vi "LatchBooleanKeyboardSimulation_Tests.vi"(11 "error in (no error)":errorcluster) -> (15 "error out":errorcluster)   [LabVIEW 2016, in "DronaTest.lvlib"]
uses:
  DronaTest.lvlib
  APIs/Stimulus/ControlValue/ValueSignalLatchBooleanString.vi
  APIs/Assert/AssertControlValue/Equal.vi
  <vilib>/addons/_JKI Toolkits/Caraya/classes/Test/Test.lvclass
  Drona.lvlib
  APIs/Assert/AssertControlValue/AssertControlValue.lvlib
  APIs/Stimulus/ControlValue/ControlValue.lvlib
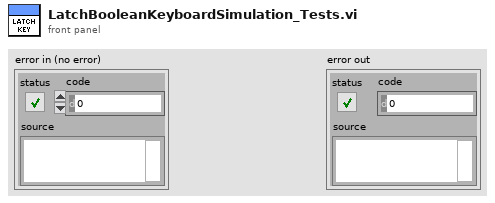
[diagram p1: front panel]
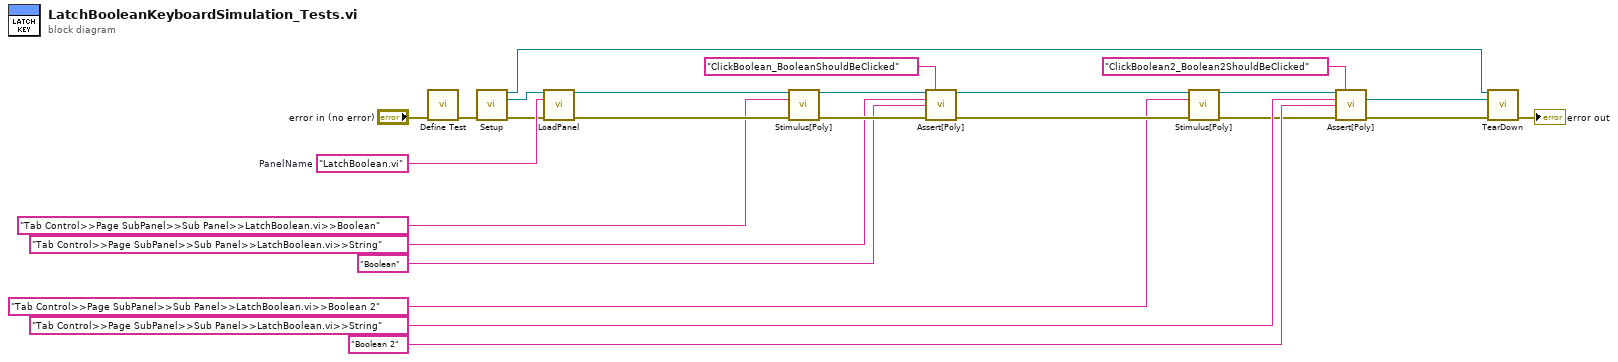
[diagram p0: block diagram]
diagram:
  w24 = "LatchBoolean.vi"  # PanelName
  n1 = call <vilib>:"Define Test.vi"("error in (no error)"="error in (no error)") -> ("error out"=w6:errorcluster)  [unwired: 10 in]
  n2 = call "Setup.vi"("error in (no error)"=w6) -> ("Application Ref"=w4:refnum<vi>, "VI out"=w2:refnum<vi>, "error out"=w3:errorcluster)  [unwired: 12 in]
  n3 = call "LoadPanel.vi"("VI in"=w2, "Panel Name"=w24, "error in (no error)"=w3) -> ("VI out"=w22:refnum<vi>, "error out"=w9:errorcluster)  [unwired: 11 in]
  n4 = call-poly "Stimulus[Poly].vi"("VI Reference In"=w22, "Control Path"="Tab Control>>Page SubPanel>>Sub Panel>>LatchBoolean.vi>>Boolean", "error in"=w9) -> ("VI Reference Out"=w21:refnum<vi>, "error out"=w23:errorcluster)  [unwired: 11 in]
  n5 = call-poly "Assert[Poly].vi"("VI Reference In"=w21, "Test Label"="ClickBoolean_BooleanShouldBeClicked" ("string"), "Control Path"="Tab Control>>Page SubPanel>>Sub Panel>>LatchBoolean.vi>>String", "Control Value"="Boolean" ("Control Path"), "Error In"=w23) -> ("VI Reference Out"=w11:refnum<vi>, "Error Out"=w12:errorcluster)  [unwired: 9 in]
  n6 = call-poly "Stimulus[Poly].vi"("VI Reference In"=w11, "Control Path"="Tab Control>>Page SubPanel>>Sub Panel>>LatchBoolean.vi>>Boolean 2", "error in"=w12) -> ("VI Reference Out"=w14:refnum<vi>, "error out"=w13:errorcluster)  [unwired: 11 in]
  n7 = call-poly "Assert[Poly].vi"("VI Reference In"=w14, "Test Label"="ClickBoolean2_Boolean2ShouldBeClicked" ("string"), "Control Path"="Tab Control>>Page SubPanel>>Sub Panel>>LatchBoolean.vi>>String", "Control Value"="Boolean 2" ("Control Path"), "Error In"=w13) -> ("VI Reference Out"=w1:refnum<vi>, "Error Out"=w10:errorcluster)  [unwired: 9 in]
  n8 = call "TearDown.vi"("Application Ref"=w4, "VI in"=w1, "error in (no error)"=w10) -> ("error out"=→"error out":errorcluster)  [unwired: 12 in]
